vi "DATE WISE.vi"(0 "Refnum in":T1, 1 "To Date":timestamp, 2 "Shift":string, 3 "Select Stakeholder":string, 4 "Select Line":string, 5 "error in (no error)":errorcluster, 6 "Form Date":timestamp, 7 "columns":string[](array[string]), 8 "total in date":string[](array[string]), 9 "STAKEHOLDER COSTANT":string="5") -> (11 "COUNT OF ARRAY":dbl, 12 "Count out":string[](array[string]), 14 "Refnum out":T1, 15 "DURATION":string[](array[string]), 16 "DURATION SUM OF ARRAY":dbl, 17 "output":string[][](array[string]), 19 "error out":errorcluster)   [LabVIEW 2017]
uses:
  <vilib>/addons/database/Connection.llb/Conn ObjectReference.ctl
  <vilib>/addons/database/NI_Database_API.lvlib
panel:
  out "Array":string[](array[string])
  out "data 2":variant[][](array[variant])
  out "Elements Found out":string[](array[string])
  out "string min  4":string[](array[string])
  out "gap leader":string[][](array[string])
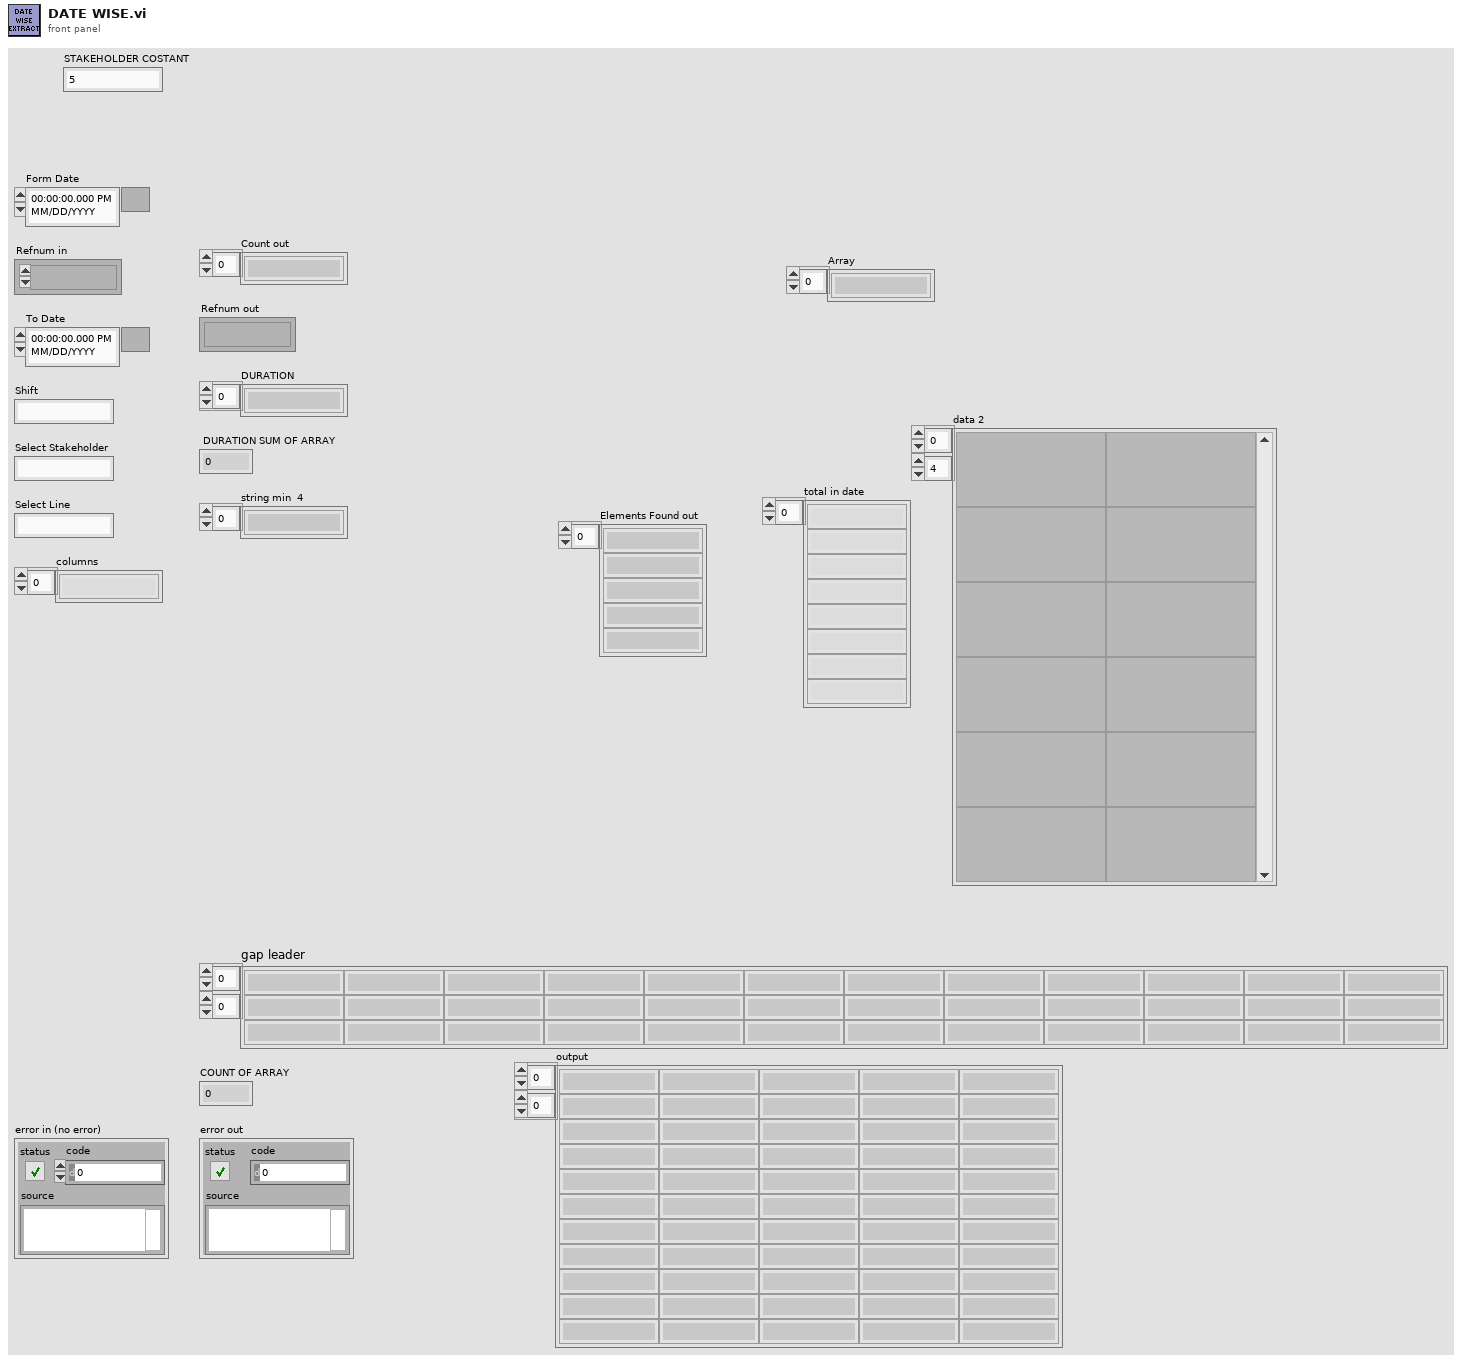
[diagram p1: front panel]
types:
  T1 = typedef "NI_Database_API.lvlib/Conn ObjectReference.ctl" = refnum<k1>
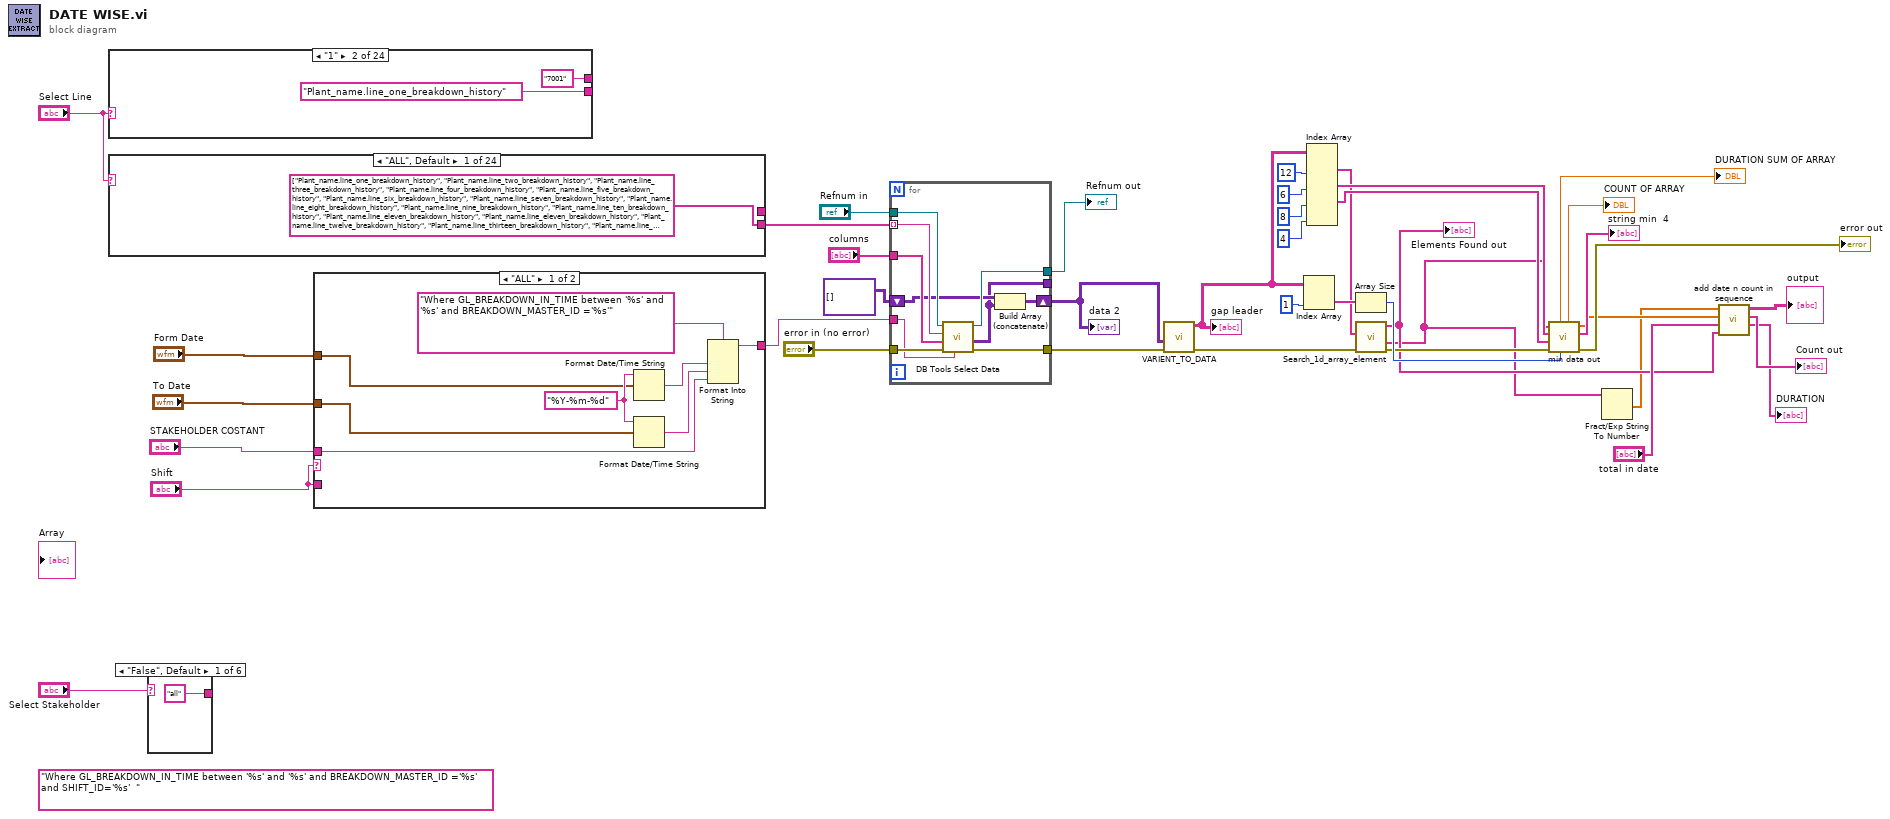
[diagram p0: block diagram]
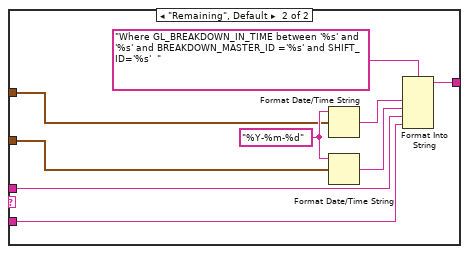
[diagram p2: hidden frame]
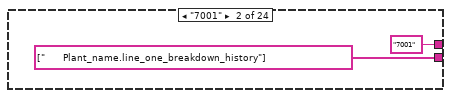
[diagram p3: hidden frame]
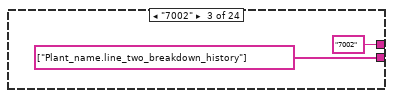
[diagram p4: hidden frame]
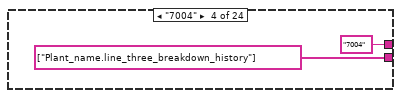
[diagram p5: hidden frame]
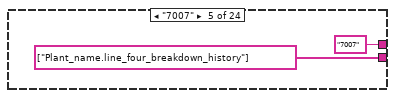
[diagram p6: hidden frame]
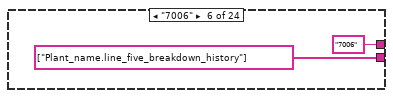
[diagram p7: hidden frame]
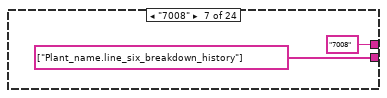
[diagram p8: hidden frame]
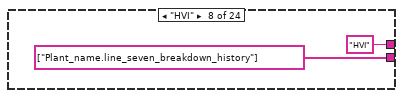
[diagram p9: hidden frame]
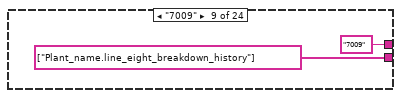
[diagram p10: hidden frame]
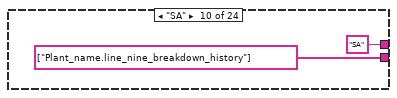
[diagram p11: hidden frame]
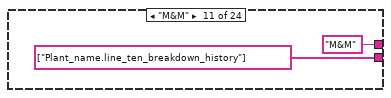
[diagram p12: hidden frame]
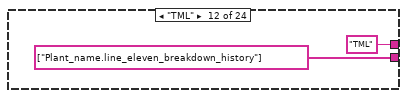
[diagram p13: hidden frame]
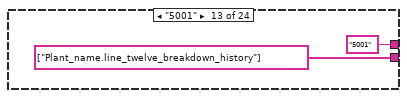
[diagram p14: hidden frame]
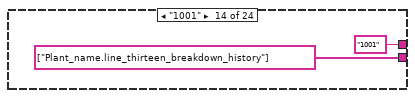
[diagram p15: hidden frame]
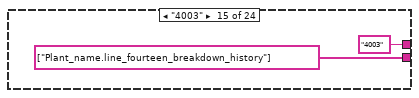
[diagram p16: hidden frame]
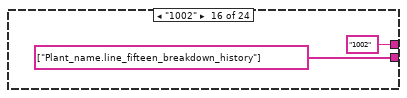
[diagram p17: hidden frame]
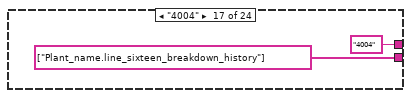
[diagram p18: hidden frame]
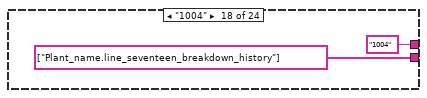
[diagram p19: hidden frame]
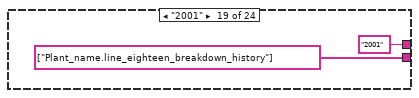
[diagram p20: hidden frame]
diagram:
  (unwired) "Where GL_BREAKDOWN_IN_TIME between '%s' and '%s' and BREAKDOWN_MASTER_ID ='%s'  and SHIFT_ID='%s'  " ("condition")
  n1 = case shown="\"1\"" "Select Line" {
    tunnel: [_ "7001" "7002" "7004" "7007" "7006" "7008" "HVI" "7009" "SA" "M&M" "TML" "5001" "1001" "4003" "1002" "4004" "1004" "2001" "3001" "2004" "3002" "3003" "4001"] -> _
    tunnel: [_ "Plant_name.line_one_breakdown_history" ("table") "Plant_name.line_two_breakdown_history" ("table") "Plant_name.line_three_breakdown_history" ("table") "Plant_name.line_four_breakdown_history" ("table") "Plant_name.line_five_breakdown_history" ("table") "Plant_name.line_six_breakdown_history" ("table") "Plant_name.line_seven_breakdown_history" ("table") "Plant_name.line_eight_breakdown_history" ("table") "Plant_name.line_nine_breakdown_history" ("table") "Plant_name.line_ten_breakdown_history" ("table") "Plant_name.line_eleven_breakdown_history" ("table") "Plant_name.line_twelve_breakdown_history" ("table") "Plant_name.line_thirteen_breakdown_history" ("table") "Plant_name.line_fourteen_breakdown_history" ("table") "Plant_name.line_fifteen_breakdown_history" ("table") "Plant_name.line_sixteen_breakdown_history" ("table") "Plant_name.line_seventeen_breakdown_history" ("table") "Plant_name.line_eighteen_breakdown_history" ("table") "Plant_name.line_nineteen_breakdown_history" ("table") "Plant_name.line_twenty_breakdown_history" ("table") "Plant_name.line_twenty_one_breakdown_history" ("table") "Plant_name.line_twenty_two_breakdown_history" ("table") "Plant_name.line_twenty_three_breakdown_history" ("table")] -> _
    frame "0", Default {
    }
    frame "1" {
    }
    frame "2" {
    }
    frame "3" {
    }
    frame "4" {
    }
    frame "5" {
    }
    frame "6" {
    }
    frame "7" {
    }
    frame "8" {
    }
    frame "9" {
    }
    frame "10" {
    }
    frame "11" {
    }
    frame "12" {
    }
    frame "13" {
    }
    frame "14" {
    }
    frame "15" {
    }
    frame "16" {
    }
    frame "17" {
    }
    frame "18" {
    }
    frame "19" {
    }
    frame "20" {
    }
    frame "21" {
    }
    frame "22" {
    }
    frame "23" {
    }
  }
  n2 = case shown="\"ALL\", Default" "Select Line" {
    tunnel: [_ "7001" "7002" "7004" "7007" "7006" "7008" "HVI" "7009" "SA" "M&M" "TML" "5001" "1001" "4003" "1002" "4004" "1004" "2001" "3001" "2004" "3002" "3003" "4001"] -> _
    tunnel: [string[] ["Plant_name.line_one_breakdown_history", "Plant_name.line_two_breakdown_history", "Plant_name.line_three_breakdown_history", "Plant_name.line_four_breakdown_history", "Plant_name.line_five_breakdown_history", "Plant_name.line_six_breakdown_history", "Plant_name.line_seven_breakdown_history", "Plant_name.line_eight_breakdown_history", "Plant_name.line_nine_breakdown_history", "Plant_name.line_ten_breakdown_history", "Plant_name.line_eleven_breakdown_history", "Plant_name.line_eleven_breakdown_history", "Plant_name.line_twelve_breakdown_history", "Plant_name.line_thirteen_breakdown_history", "Plant_name.line_fourteen_breakdown_history", "Plant_name.line_fifteen_breakdown_history", "Plant_name.line_sixteen_breakdown_history", "Plant_name.line_seventeen_breakdown_history", "Plant_name.line_eighteen_breakdown_history", "Plant_name.line_nineteen_breakdown_history", "Plant_name.line_twenty_breakdown_history", "Plant_name.line_twenty_one_breakdown_history", "Plant_name.line_twenty_two_breakdown_history", "Plant_name.line_twenty_three_breakdown_history"] string[] ["      Plant_name.line_one_breakdown_history"] string[] ["Plant_name.line_two_breakdown_history"] string[] ["Plant_name.line_three_breakdown_history"] string[] ["Plant_name.line_four_breakdown_history"] string[] ["Plant_name.line_five_breakdown_history"] string[] ["Plant_name.line_six_breakdown_history"] string[] ["Plant_name.line_seven_breakdown_history"] string[] ["Plant_name.line_eight_breakdown_history"] string[] ["Plant_name.line_nine_breakdown_history"] string[] ["Plant_name.line_ten_breakdown_history"] string[] ["Plant_name.line_eleven_breakdown_history"] string[] ["Plant_name.line_twelve_breakdown_history"] string[] ["Plant_name.line_thirteen_breakdown_history"] string[] ["Plant_name.line_fourteen_breakdown_history"] string[] ["Plant_name.line_fifteen_breakdown_history"] string[] ["Plant_name.line_sixteen_breakdown_history"] string[] ["Plant_name.line_seventeen_breakdown_history"] string[] ["Plant_name.line_eighteen_breakdown_history"] string[] ["Plant_name.line_nineteen_breakdown_history"] string[] ["Plant_name.line_twenty_breakdown_history"] string[] ["Plant_name.line_twenty_one_breakdown_history"] string[] ["Plant_name.line_twenty_two_breakdown_history"] string[] ["Plant_name.line_twenty_three_breakdown_history"]] -> w22
    frame "ALL", Default {
    }
    frame "7001" {
    }
    frame "7002" {
    }
    frame "7004" {
    }
    frame "7007" {
    }
    frame "7006" {
    }
    frame "7008" {
    }
    frame "HVI" {
    }
    frame "7009" {
    }
    frame "SA" {
    }
    frame "M&M" {
    }
    frame "TML" {
    }
    frame "5001" {
    }
    frame "1001" {
    }
    frame "4003" {
    }
    frame "1002" {
    }
    frame "4004" {
    }
    frame "1004" {
    }
    frame "2001" {
    }
    frame "3001" {
    }
    frame "2004" {
    }
    frame "3002" {
    }
    frame "3003" {
    }
    frame "4001" {
    }
  }
  n3 = case shown="\"False\", Default" "Select Stakeholder" {
    tunnel: ["all" "1" "2" "3" "4" "5"] -> _
    frame "False", Default {
    }
    frame "Logistics" {
    }
    frame "Maintenance" {
    }
    frame "Quality" {
    }
    frame "Production" {
    }
    frame "Gap Leader" {
    }
  }
  n4 = case shown="\"ALL\"" "Shift" {
    tunnel: "Form Date" -> [w143 w152]
    tunnel: "To Date" -> [w142 w151]
    tunnel: "Shift" -> [_ w149]
    tunnel: [w141 w150] -> w16
    tunnel: "STAKEHOLDER COSTANT" -> [w140 w148]
    frame "ALL" {
      w147 = "%Y-%m-%d" ("time format string (%c)")
      n5 = Format Date/Time String(time format string (%c)=w147, seconds (now)=w143) -> (date/time string=w145:string)  [unwired: 1 in]
      n6 = Format Date/Time String(time format string (%c)=w147, seconds (now)=w142) -> (date/time string=w146:string)  [unwired: 1 in]
      n7 = Format Into String(format string="Where GL_BREAKDOWN_IN_TIME between '%s' and '%s' and BREAKDOWN_MASTER_ID ='%s'" ("condition"), w145, w146, w140) -> (resulting string=w141:string)  [unwired: 2 in, 1 out]
    }
    frame "Remaining", Default {
      w156 = "%Y-%m-%d" ("time format string (%c)")
      n8 = Format Date/Time String(time format string (%c)=w156, seconds (now)=w152) -> (date/time string=w154:string)  [unwired: 1 in]
      n9 = Format Date/Time String(time format string (%c)=w156, seconds (now)=w151) -> (date/time string=w155:string)  [unwired: 1 in]
      n10 = Format Into String(format string="Where GL_BREAKDOWN_IN_TIME between '%s' and '%s' and BREAKDOWN_MASTER_ID ='%s' and SHIFT_ID='%s'  " ("condition"), w154, w155, w148, w149) -> (resulting string=w150:string)  [unwired: 2 in, 1 out]
    }
  }
  n11 = for {
    tunnel: w22 -> [w164] mode=indexing
    tunnel: [w158] -> _
    tunnel: "columns" -> [w160]
    tunnel: w16 -> [w161]
    tunnel: "error in (no error)" -> [w163]
    tunnel: [w162] -> w12
    tunnel: "Refnum in" -> [w166]
    tunnel: [w165] -> w13
    shift-right: [w157] -> w14
    shift-left: variant[][] [] ("data") -> [w159]
    n12 = call <vilib>:"DB Tools Select Data.vi"("condition"=w161, "error in (no error)"=w163, "columns"=w160, "table"=w164, "connection reference"=w166) -> ("error out"=w162:errorcluster, "data"=w158:variant[][], "connection reference out"=w165:T1)  [unwired: 1 in]
    n13 = Build Array (concatenate)(w159, w158) -> (w157:variant[][])
  }
  "Refnum out" <- w13
  "data 2" <- w14
  n14 = call "VARIENT_TO_DATA.vi"("data"=w14, "error in (no error)"=w12) -> ("Table"=w36:string[][], "error out"=w35:errorcluster)  [unwired: 7 in]
  "gap leader" <- w36
  n15 = Index Array(array=w36, index (col)=1 ("disabled index (col)")) -> (element=w31:string[])  [unwired: 1 in]
  n16 = Index Array(array=w36, index (col) #1=12 ("index (row)"), index (col) #2=6 ("index (col)"), index (col) #3=8 ("index (col)"), index (col) #4=4 ("index (col)")) -> (element #1=w26:string[], element #2=w32:string[], element #3=w33:string[])  [unwired: 4 in, 1 out]
  n17 = Array Size(array=w31) -> (size(s)=w40:i32)
  n18 = call "Search_1d_array_element.vi"("error in (no error)"=w35, "BD Date"=w26) -> ("error out"=w34:errorcluster, "Count out"=w5:string[], "Elements Found out"=w6:string[])  [unwired: 5 in]
  "Elements Found out" <- w6
  n19 = call "min data out.vi"("Numeric"=w40, "error in (no error)"=w34, "out time"=w33, "in time"=w32, "Count in"=w5) -> ("error out"=→"error out":errorcluster, "string min"=→"string min  4":string[], "duration"=w7:dbl[], "COUNT OF ARRAY"=→"COUNT OF ARRAY":dbl, "DURATION SUM OF ARRAY"=→"DURATION SUM OF ARRAY":dbl)  [unwired: 2 in]
  n20 = Fract/Exp String To Number(string=w5) -> (number=w4:dbl[])  [unwired: 3 in, 1 out]
  n21 = call "add date n count in sequence.vi"("find date"=w6, "total date"="total in date", "duration"=w7, "count"=w4) -> ("DURATION"=→"DURATION":string[], "COUNT"=→"Count out":string[], "appended array"=→"output":string[][])  [unwired: 5 in]
